vi "State_Machine.vi"(8 "error in (no error)":errorcluster caption="entrée d'erreur (pas d'erreur)", 11 "Flash_AVRDUDE en entrée":refnum<class "Flash_Epox.lvclass">) -> (0 "error out":errorcluster caption="sortie d'erreur", 2 "Json_String":string, 3 "Flash_AVRDUDE en sortie":refnum<class "Flash_Epox.lvclass">)   [LabVIEW 2020, in "Library Test.lvlib" / "Flash_Epox.lvclass"]
uses:
  Flash_Epox.lvclass
  C:/Users/ngarcin/OneDrive - Altyor/Standard TB/Class/Test/Test (Default)/Test (Default).lvclass
  Flash_Epox.lvclass/Flash_Epox.ctl
panel:
  out "String In progress":string
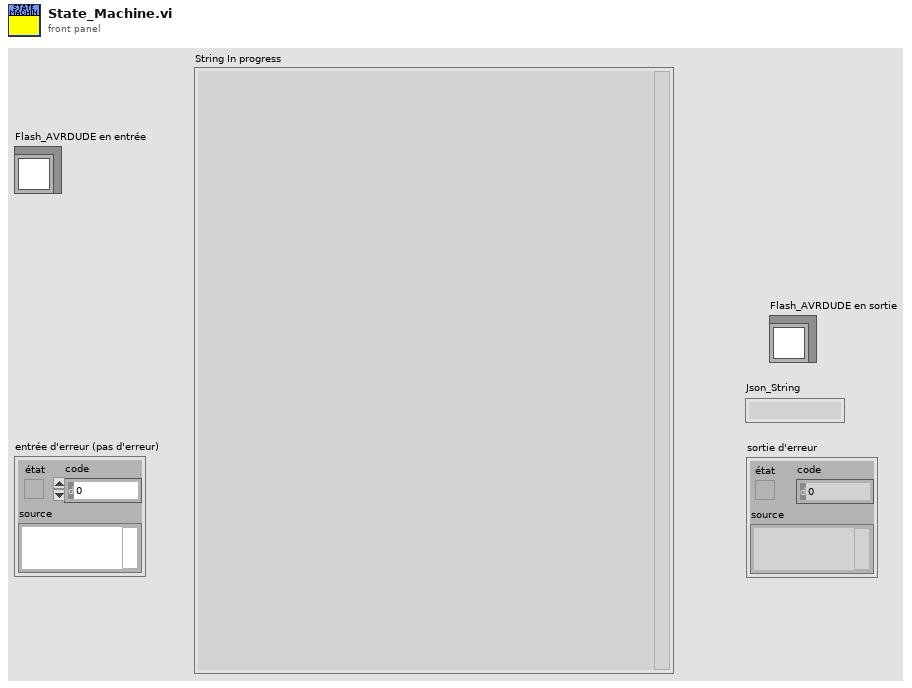
[diagram p1: front panel]
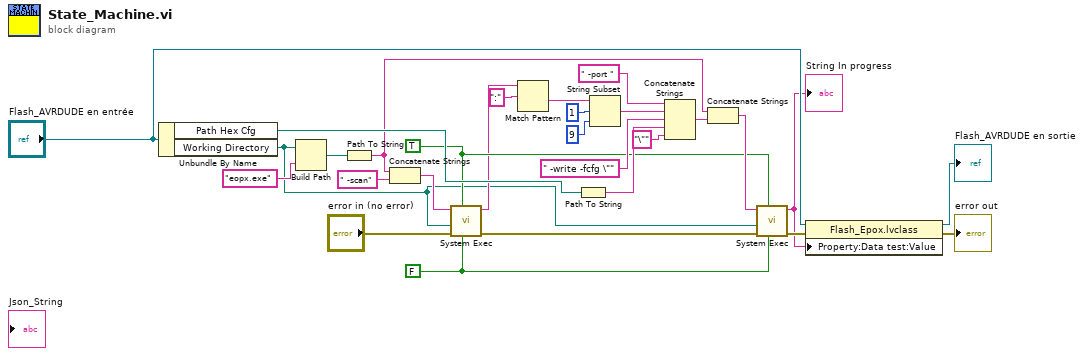
[diagram p0: block diagram]
diagram:
  w11 = TRUE ("wait until completion? (T)")
  w10 = FALSE ("run minimized? (F)")
  n1 = Unbundle By Name("Flash_AVRDUDE en entrée") -> ("Path Hex Cfg"=w23:path, "Working Directory"=w1:path)
  n2 = Build Path(base path=w1, name or relative path="eopx.exe" ("nom ou chemin relatif")) -> (appended path=w28:path)
  n3 = Path To String(path=w28) -> (string=w14:string)
  n4 = Concatenate Strings(w14, " -scan" ("chaîne")) -> (w12:string)
  n5 = call <vilib>:"System Exec.vi"("run minimized? (F)"=w10, "wait until completion? (T)"=w11, "error in (no error)"="error in (no error)", "working directory"=w1, "command line"=w12) -> ("error out"=w15:errorcluster, "standard output"=w3:string)  [unwired: 3 in, 2 out]
  n6 = Match Pattern(string=w3, regular expression=":" ("expression régulière")) -> (after substring=w8:string)  [unwired: 1 in, 3 out]
  n7 = Path To String(path=w23) -> (string=w18:string)
  n8 = String Subset(string=w8, offset (0)=1, length (rest)=9 ("longueur (reste)")) -> (substring=w5:string)
  n9 = Concatenate Strings(" -port " ("FileName"), w5, " -write -fcfg \"" ("FileName"), w18, "\"" ("chaîne")) -> (w25:string)
  n10 = Concatenate Strings(w14, w25) -> (w24:string)
  n11 = call <vilib>:"System Exec.vi"("run minimized? (F)"=w10, "wait until completion? (T)"=w11, "error in (no error)"=w15, "working directory"=w1, "command line"=w24) -> ("error out"=w19:errorcluster, "standard output"=w2:string)  [unwired: 3 in, 2 out]
  "String In progress" <- w2
  n12 = property class="Flash_Epox.lvclass"(reference="Flash_AVRDUDE en entrée", error in=w19, "Property:Data test:Value"=w2) -> (reference out=→"Flash_AVRDUDE en sortie":refnum<class "Flash_Epox.lvclass">, error out=→"error out":errorcluster)
